vi "Word_New_Page.vi"(0 "Word._Document":refnum<k7>, 7 "bookmark (Word)":string, 11 "error in":errorcluster) -> (15 "error out":errorcluster)   [LabVIEW 2020, in "NI_ReportGenerationToolkit.lvlib"]
uses:
  <vilib>/addons/_office/NI_ReportGenerationToolkit.lvlib
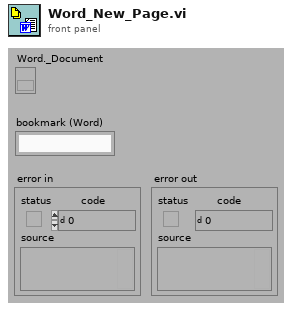
[diagram p1: front panel]
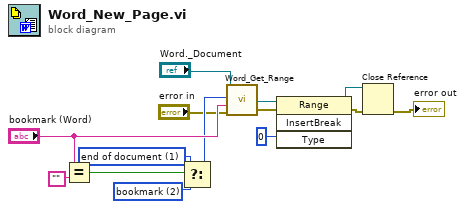
[diagram p0: block diagram]
diagram:
  w10 = u16 1 items=["begining of document", "end of document", "bookmark", "custom"] ("Insertion point")
  w9 = u16 2 items=["begining of document", "end of document", "bookmark", "custom"] ("Insertion point")
  n1 = Equal?(x="bookmark (Word)", y="") -> (x = y?=w11:bool)
  n2 = Select(t=w10, s=w11, f=w9) -> (s? t:f=w13:u16)
  n3 = call <vilib>:"Word_Get_Range.vi"("error in"="error in", "bookmark name"="bookmark (Word)", "insertion point"=w13, "document in"="Word._Document") -> ("error out (no error)"=w4:errorcluster, "range"=w2:refnum<k7>)  [unwired: 2 in, 4 out]
  n4 = invoke class="Range" method="InsertBreak"(reference=w2, error in=w4, "Type"=0) -> (reference out=w6:refnum<k7>, error out=w5:errorcluster)  [unwired: 1 in, 2 out]
  n5 = Close Reference(reference=w6, error in (no error)=w5) -> (error out=→"error out":errorcluster)
